vi "BRig_Host__Loop_Producer__UploadClosedLoop_recordCmdList__v2.vi"(5 "input_newData":i64[][](array[numeric]), 7 "input_n":i32) -> ()   [LabVIEW 2014]
uses:
  <vilib>/Utility/file.llb/Read From Spreadsheet File (I64).vi
  <vilib>/Utility/file.llb/Write To Spreadsheet File (I64).vi
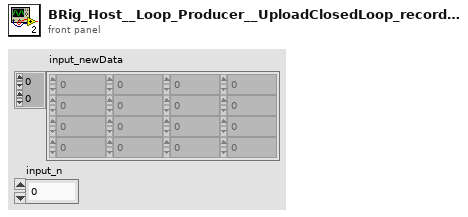
[diagram p1: front panel]
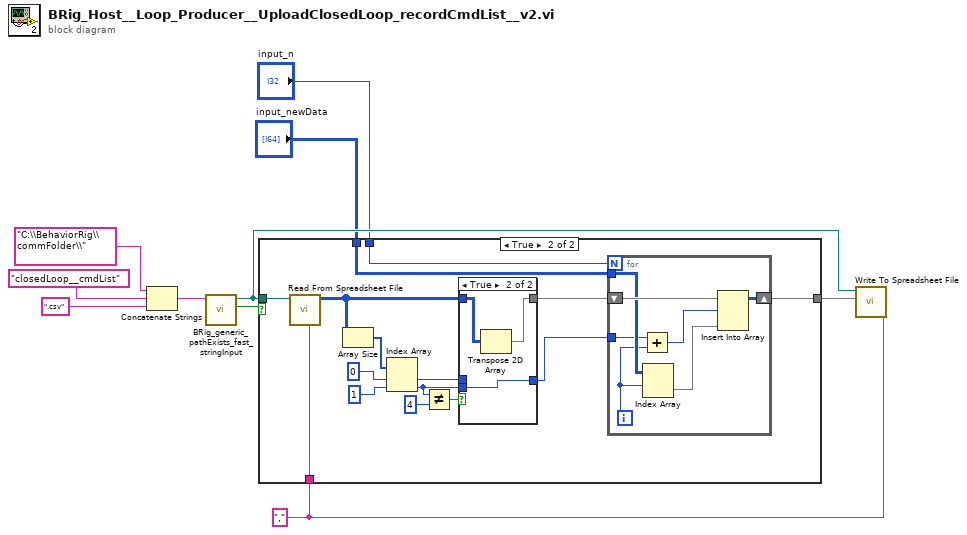
[diagram p0: block diagram]
diagram:
  w2 = "," ("delimiter (\\t)")
  n1 = Concatenate Strings("C:\\BehaviorRig\\commFolder\\", "closedLoop__cmdList" ("string"), ".csv" ("string")) -> (w7:string)
  n2 = call "BRig_generic_pathExists_fast_stringInput.vi"("input_filePath"=w7) -> ("output_Iexist"=w1:bool, "output_filePath"=w6:path)  [unwired: 8 in, 1 out]
  n3 = case shown="True" w1 {
    tunnel: w6 -> [_ w26]
    tunnel: "input_newData" -> [w11 w16]
    tunnel: [w11 w13] -> w4
    tunnel: "input_n" -> [_ w17]
    tunnel: w2 -> [_ w12]
    frame False {
    }
    frame True {
      n4 = call-poly <vilib>:"Read From Spreadsheet File.vi"("delimiter (\\t)"=w12, "file path (dialog if empty)"=w26) -> ("all rows"=w20:i64[][])  [unwired: 5 in, 4 out]
      n5 = Array Size(array=w20) -> (size(s)=w25:i32[])
      n6 = Index Array(array=w25, index #1=0 ("index"), index #2=1 ("index")) -> (element #1=w18:i32, element #2=w19:i32)
      n7 = Not Equal?(x=w19, y=4) -> (x != y?=w21:bool)
      n8 = case shown="True" w21 {
        tunnel: w20 -> [w35 w38]
        tunnel: [w35 w37] -> w15
        tunnel: w19 -> [_ w36]
        tunnel: [w34 w36] -> w14
        tunnel: w18 -> [w34 _]
        frame False {
        }
        frame True {
          n9 = Transpose 2D Array(2D array=w38) -> (transposed array=w37:i64[][])
        }
      }
      n10 = for {
        N: w17 -> [_]
        tunnel: w16 -> [w31]
        shift-right: [w33] -> w13
        shift-left: w15 -> [w32]
        tunnel: w14 -> [w29]
        i -> [w30]
        n11 = Add(x=w29, y=w30) -> (x+y=w28:i32)
        n12 = Index Array(array=w31, index (row)=w30) -> (element=w27:i64[])  [unwired: 1 in]
        n13 = Insert Into Array(array=w32, index (row)=w28, new element=w27) -> (w33:i64[][])  [unwired: 1 in]
      }
    }
  }
  n14 = call-poly <vilib>:"Write To Spreadsheet File.vi"("delimiter (\\t)"=w2, "2D data"=w4, "file path (dialog if empty)"=w6) -> ()  [unwired: 5 in, 1 out]
